vi "Configure Offset And Limits List (Spectrum Emissions Mask - Relative And Absolute Limits).vi"(0 "VISA resource name":refnum<visa-resource-name>, 1 "Auto Relative":u16[](array[ring])=[0, 0] items=["Couple", "Man"], 2 "Relative Start Values":dbl[](array[numeric])=[-30.0, -30.0] format="%#.6g", 3 "Relative Stop Values":dbl[](array[numeric])=[-30.0, -30.0] format="%#.6g", 5 "Auto Absolute":u16[](array[ring])=[0, 0] items=["Couple", "Man"], 7 "Absolute Start Values":dbl[](array[numeric])=[-14.0, -14.0] format="%#.6g", 9 "Absolute Stop Values":dbl[](array[numeric])=[-14.0, -14.0] format="%#.6g", 11 "error in (no error)":errorcluster, 12 "Fail Mask":u16[](array[ring])=[0, 0] items=["Absolute", "Relative", "Absolute And Relative", "Absolute Or Relative"]) -> (4 "VISA resource name out":refnum<visa-resource-name>, 15 "error out":errorcluster)   [LabVIEW 2014, in "Agilent ESA PSA Series.lvlib"]
doc: "Sets the start and stop frequency for the relative limit of a specific offset for spectrum analyzer spectrum emission mask measurements."
uses:
  Agilent ESA PSA Series.lvlib
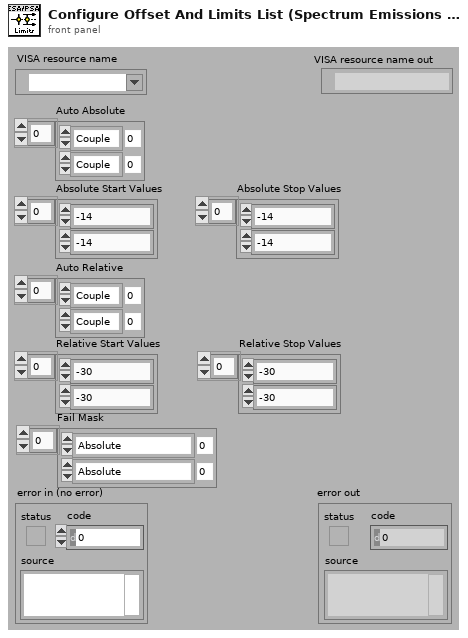
[diagram p1: front panel]
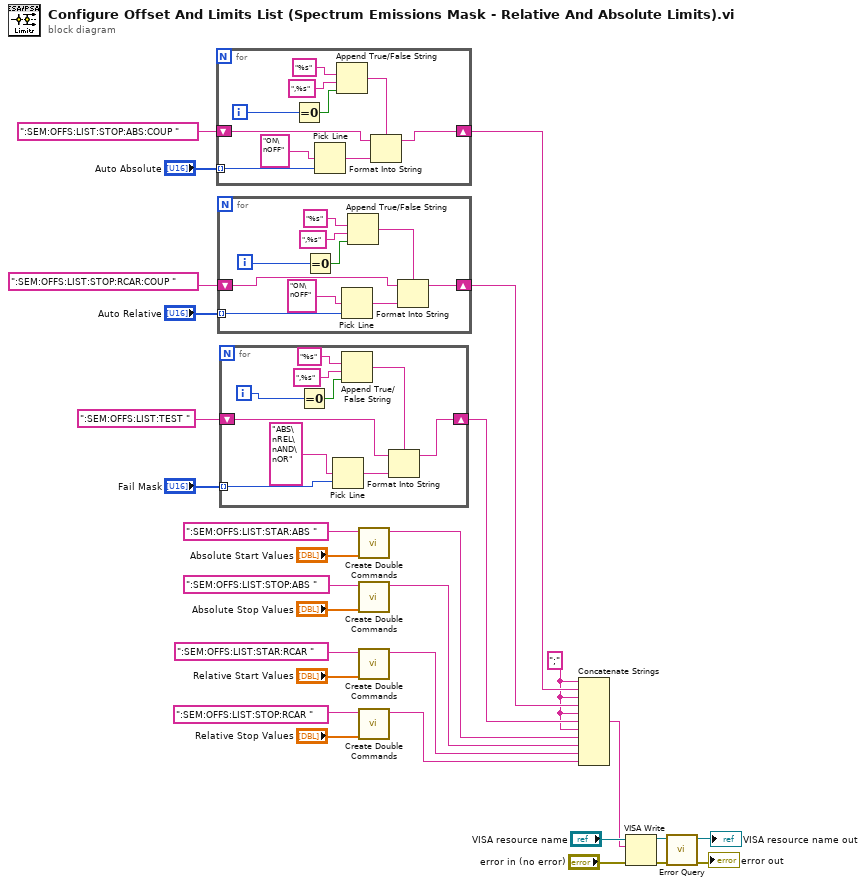
[diagram p0: block diagram]
diagram:
  w13 = ";" ("string")
  n1 = for {
    tunnel: "Auto Absolute" -> [w39] mode=indexing
    shift-right: [w37] -> w15
    shift-left: ":SEM:OFFS:LIST:STOP:ABS:COUP " -> [w38]
    i -> [w30]
    n2 = Equal To 0?(x=w30) -> (x = 0?=w34:bool)
    n3 = Pick Line(multi-line string="ON\nOFF" ("format string"), line index=w39) -> (output string=w32:string)  [unwired: 1 in]
    n4 = Append True/False String(1:w34, 2:",%s" ("format string"), 3:"%s" ("format string")) -> (0:w31:string)  [unwired: 1 in]
    n5 = Format Into String(format string=w31, initial string=w38, w32) -> (resulting string=w37:string)  [unwired: 1 in, 1 out]
  }
  n6 = for {
    tunnel: "Auto Relative" -> [w49] mode=indexing
    shift-right: [w47] -> w16
    shift-left: ":SEM:OFFS:LIST:STOP:RCAR:COUP " -> [w48]
    i -> [w40]
    n7 = Equal To 0?(x=w40) -> (x = 0?=w44:bool)
    n8 = Pick Line(multi-line string="ON\nOFF" ("format string"), line index=w49) -> (output string=w45:string)  [unwired: 1 in]
    n9 = Append True/False String(1:w44, 2:",%s" ("format string"), 3:"%s" ("format string")) -> (0:w41:string)  [unwired: 1 in]
    n10 = Format Into String(format string=w41, initial string=w48, w45) -> (resulting string=w47:string)  [unwired: 1 in, 1 out]
  }
  n11 = for {
    tunnel: "Fail Mask" -> [w59] mode=indexing
    shift-right: [w57] -> w17
    shift-left: ":SEM:OFFS:LIST:TEST " -> [w58]
    i -> [w50]
    n12 = Equal To 0?(x=w50) -> (x = 0?=w52:bool)
    n13 = Pick Line(multi-line string="ABS\nREL\nAND\nOR" ("format string"), line index=w59) -> (output string=w56:string)  [unwired: 1 in]
    n14 = Append True/False String(1:w52, 2:",%s" ("format string"), 3:"%s" ("format string")) -> (0:w51:string)  [unwired: 1 in]
    n15 = Format Into String(format string=w51, initial string=w58, w56) -> (resulting string=w57:string)  [unwired: 1 in, 1 out]
  }
  n16 = call "Create Double Commands.vi"("Double Values"="Absolute Start Values", "Commands"=":SEM:OFFS:LIST:STAR:ABS ") -> ("Result"=w4:string)  [unwired: 9 in]
  n17 = call "Create Double Commands.vi"("Double Values"="Absolute Stop Values", "Commands"=":SEM:OFFS:LIST:STOP:ABS ") -> ("Result"=w3:string)  [unwired: 9 in]
  n18 = call "Create Double Commands.vi"("Double Values"="Relative Start Values", "Commands"=":SEM:OFFS:LIST:STAR:RCAR ") -> ("Result"=w2:string)  [unwired: 9 in]
  n19 = call "Create Double Commands.vi"("Double Values"="Relative Stop Values", "Commands"=":SEM:OFFS:LIST:STOP:RCAR ") -> ("Result"=w1:string)  [unwired: 9 in]
  n20 = Concatenate Strings(w13, w15, w13, w16, w13, w17, w13, w4, w3, w2, w1) -> (w14:string)
  n21 = VISA Write(VISA resource name="VISA resource name", write buffer=w14, error in (no error)="error in (no error)") -> (VISA resource name out=w23:refnum<visa-resource-name>, error out=w22:errorcluster)  [unwired: 1 out]
  n22 = call "Error Query.vi"("error in (no error)"=w22, "VISA resource name"=w23) -> ("error out"=→"error out":errorcluster, "VISA resource name out"=→"VISA resource name out":refnum<visa-resource-name>)  [unwired: 6 in, 2 out]
